vi "Shift_Control.vi"(0 "right_whlspd":dbl, 1 "left_whlspd":dbl, 2 "Joystick_Y":dbl, 3 "high_throt_thresh":dbl=75.0 format="%#_13g", 4 "low_throt_thresh":dbl=20.0 format="%#_13g", 5 "auto_ds_spd_hiload":dbl, 6 "auto_us_en":bool=TRUE, 7 "auto_us_spd":dbl=60000.0, 8 "auto_ds_en":bool=TRUE, 9 "manual_shift_req":bool) -> (14 "High_Gear_Cmd":bool)   [LabVIEW 2015]
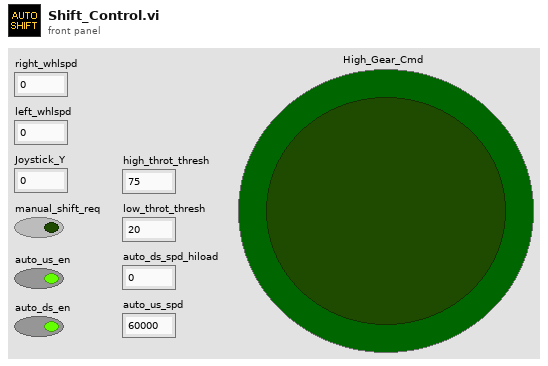
[diagram p1: front panel]
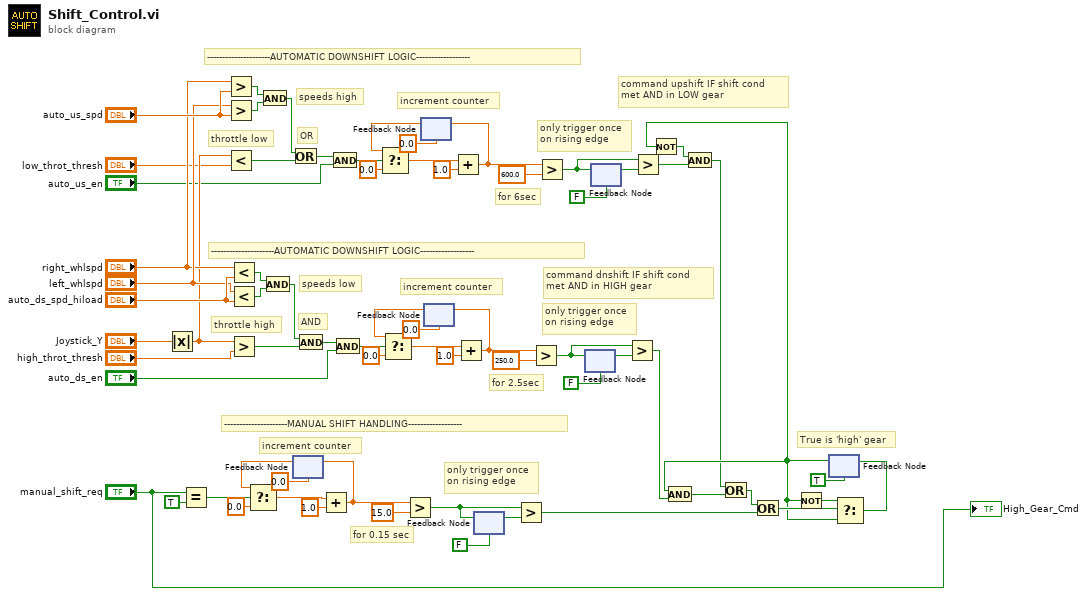
[diagram p0: block diagram]
diagram:
  # "---------------------MANUAL SHIFT HANDLING------------------"
  # "command dnshift IF shift cond \nmet AND in HIGH gear"
  # "command upshift IF shift cond \nmet AND in LOW gear"
  # "AND"
  # "OR"
  # "---------------------AUTOMATIC DOWNSHIFT LOGIC------------------"
  # "---------------------AUTOMATIC DOWNSHIFT LOGIC------------------"
  # "only trigger once\non rising edge"
  # "for 6sec"
  # "increment counter"
  # "throttle low"
  # "speeds high"
  # "True is 'high' gear"
  # "only trigger once\non rising edge"
  # "for 0.15 sec"
  # "increment counter"
  # "only trigger once\non rising edge"
  # "for 2.5sec"
  # "increment counter"
  # "throttle high"
  # "speeds low"
  n1 = Absolute Value(x="Joystick_Y") -> (abs(x)=w14:dbl)
  n2 = Equal?(x="manual_shift_req", y=TRUE) -> (x = y?=w49:bool)
  n3 = Greater?(x="right_whlspd", y="auto_us_spd") -> (0:w32:bool)
  n4 = Greater?(x="left_whlspd", y="auto_us_spd") -> (0:w33:bool)
  n5 = Less?(x=w14, y="low_throt_thresh") -> (x < y?=w31:bool)
  n6 = Less?(x="right_whlspd", y="auto_ds_spd_hiload") -> (x < y?=w66:bool)
  n7 = Less?(x="left_whlspd", y="auto_ds_spd_hiload") -> (x < y?=w67:bool)
  n8 = Greater?(x=w14, y="high_throt_thresh") -> (0:w64:bool)
  n9 = And(x=w32, y=w33) -> (x .and. y?=w30:bool)
  n10 = And(x=w66, y=w67) -> (x .and. y?=w63:bool)
  n11 = Or(x=w30, y=w31) -> (x .or. y?=w18:bool)
  n12 = feedback #1(0.0) -> (w46:dbl)
  n13 = Select(t=w46, s=w49, f=0.0) -> (s? t:f=w45:dbl)
  n14 = And(x=w63, y=w64) -> (x .and. y?=w36:bool)
  n15 = Add(x=w45, y=1.0) -> (x+y=w47:dbl)
  n16 = feedback-in #1(w47) -> ()
  n17 = And(x=w18, y="auto_us_en") -> (x .and. y?=w19:bool)
  n18 = And(x=w36, y="auto_ds_en") -> (x .and. y?=w37:bool)
  n19 = Greater?(x=w47, y=15.0) -> (0:w3:bool)
  n20 = feedback #2(0.0) -> (w20:dbl)
  n21 = Select(t=w20, s=w19, f=0.0) -> (s? t:f=w22:dbl)
  n22 = feedback #3(0.0) -> (w42:dbl)
  n23 = Select(t=w42, s=w37, f=0.0) -> (s? t:f=w44:dbl)
  n24 = Add(x=w22, y=1.0) -> (x+y=w21:dbl)
  n25 = feedback-in #2(w21) -> ()
  n26 = Add(x=w44, y=1.0) -> (x+y=w43:dbl)
  n27 = feedback-in #3(w43) -> ()
  n28 = feedback #4(FALSE) -> (w5:bool)
  n29 = feedback-in #4(w3) -> ()
  n30 = Greater?(x=w3, y=w5) -> (0:w2:bool)
  n31 = Greater?(x=w43, y=250.0) -> (0:w58:bool)
  n32 = Greater?(x=w21, y=600.0) -> (0:w25:bool)
  n33 = feedback #5(FALSE) -> (w57:bool)
  n34 = feedback-in #5(w58) -> ()
  n35 = feedback #6(FALSE) -> (w24:bool)
  n36 = feedback-in #6(w25) -> ()
  n37 = Greater?(x=w58, y=w57) -> (0:w38:bool)
  n38 = Greater?(x=w25, y=w24) -> (0:w11:bool)
  n39 = feedback #7(TRUE) -> (w10:bool)
  n40 = Not(x=w10) -> (.not. x?=w9:bool)
  n41 = And(x=w10, y=w38) -> (x .and. y?=w7:bool)
  n42 = And(x=w9, y=w11) -> (x .and. y?=w6:bool)
  n43 = Or(x=w6, y=w7) -> (x .or. y?=w8:bool)
  n44 = Or(x=w8, y=w2) -> (x .or. y?=w39:bool)
  n45 = Not(x=w10) -> (.not. x?=w40:bool)
  n46 = Select(t=w40, s=w39, f=w10) -> (s? t:f=w41:bool)
  n47 = feedback-in #7(w41) -> ()
  "High_Gear_Cmd" <- "manual_shift_req"
